vi "Event Wait Data.vi"(8 "error in (no error)":errorcluster, 11 "Event DVR in":refnum<data-value>) -> (0 "error out":errorcluster, 2 "Data out":refnum<data-value>, 3 "Event DVR out":refnum<data-value>)   [LabVIEW 2010, in "MDSplus.lvlib"]
doc: "Return data received last."
uses:
  <vilib>/MDSplus/Library/MDSplus.lvlib
  <vilib>/MDSplus/Classes/Event_Class/Event.lvclass
  <vilib>/MDSplus/Classes/Data_Class/Data.lvclass
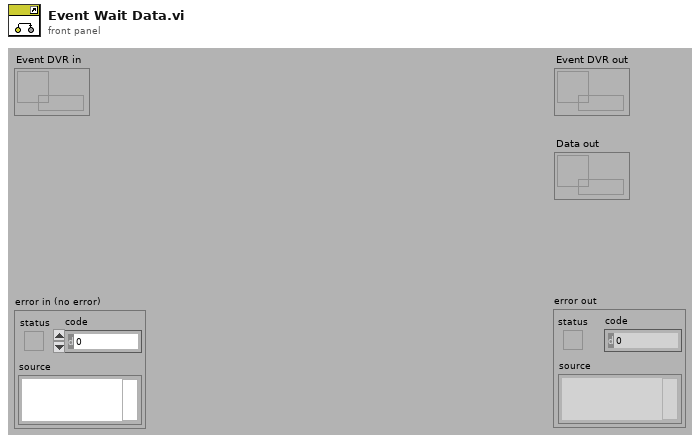
[diagram p1: front panel]
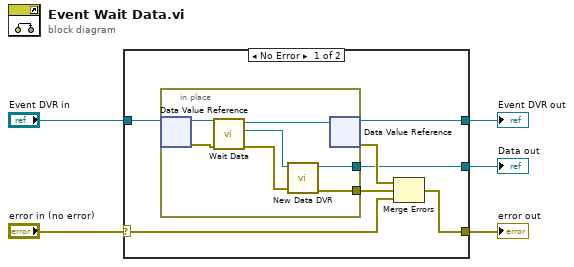
[diagram p0: block diagram]
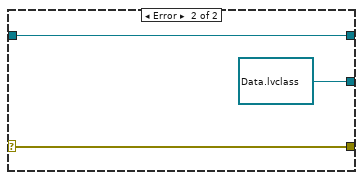
[diagram p2: hidden frame]
diagram:
  n1 = case shown="No Error" "error in (no error)" {
    selector: "error in (no error)" -> [w11 w22]
    tunnel: "Event DVR in" -> [w12 w21]
    tunnel: [w8 w22] -> w5
    tunnel: [w9 w21] -> w2
    tunnel: [w6 refnum<data-value> refnum ("Data DVR")] -> w1
    frame No Error {
      n2 = in-place {
        in-place-border: [w19] -> w6
        in-place-border: [w18] -> w7
        n3 = in-place-dvr #1(w12) -> (w16:refnum<class "Event.lvclass">, w17:errorcluster)
        n4 = call-dynamic "Wait Data.vi"("error in (no error)"=w17, "Event in"=w16) -> ("error out"=w13:errorcluster, "Data out"=w14:refnum<class "Data.lvclass">, "Event out"=w15:refnum<class "Event.lvclass">)  [unwired: 7 in]
        n5 = call <vilib>:"New Data DVR.vi"("error in (no error)"=w13, "Data in"=w14) -> ("error out"=w18:errorcluster, "Data DVR out"=w19:refnum<data-value>)  [unwired: 8 in]
        n6 = in-place-dvr #1(w15) -> (w9:refnum<data-value>, w10:errorcluster)
      }
      n7 = Merge Errors(w10, w7, w11) -> (w8:errorcluster)
    }
    frame Error {
    }
  }
  "error out" <- w5
  "Event DVR out" <- w2
  "Data out" <- w1
